vi "DAQmxDigitalOutput_2019-11-01.vi"() -> ()   [LabVIEW 2015]
uses:
  <vilib>/Analysis/baseanly.llb/Mean (DBL).vi
  <vilib>/DAQmx/create/channels.llb/DAQmx Create Channel (CO-Pulse Generation-Time).vi
  <vilib>/DAQmx/configure/timing.llb/DAQmx Timing (Implicit).vi
  MVCAMSDK.dll
  <vilib>/Analysis/NI_AALBase.lvlib
  <vilib>/Analysis/NI_AAL_SigProc.lvlib
panel:
  out "相对误差":dbl=0.8988653041973323
  out "mean":dbl=15.208009079636986 caption="泰伯距离均值Z" format="%0.2f"
  in  "光栅常数d":dbl=0.09854
  in  "error in 2":errorcluster caption="错误输入"
  in  "data 2":bool[](array[boolean])=[TRUE]
  out "测量得到的波长":dbl=638.4880196449607
  out "泰伯距离数值":dbl[](array[numeric])=[15.393849374426454, 15.239052716055017, 15.197063981826837, 15.002070246239633]
  out "移动次数":dbl=1.0
  out "Locations":dbl[](array[numeric])=[10.438621227921368, 25.832470602347822, 41.07152331840284, 56.268587300229676, 71.27065754646931] caption="上面图像曲线波峰位置"
  out "光强图":u8[](graph)=[255, 255, 255, 255, 255, 255, 255, 255, 255, 154, 43, 20, 23, 22, 53, 146, 167, 169, 232, 255, 255, 255, 255, 255, 203, 166, 115, 72, 50, 24, 17, 38, 118, 114, 190, 255, 255, 255, 255, 255, 255, 255, 255, 233, 255, 216, 118, 34, 16, 17, 18, 55, 150, 246, 222, 224, 255, 255, 255, 255, 255, 255, 150, 104, 77, 71, 41, 22, 45, 119, 116, 218, 255, 255, 255, 255, 255, 255, 255, 255, 241, 255, 255, 174, 87, 33, 17, 18, 43, 114, 155, 143, 170, 255, 255, 255, 255, 255, 255, 198, 155, 125, 91, 53, 22, 27, 94, 64, 126, 248, 255, 255, 255, 255, 255, 255, 255, 238, 232, 255, 240, 144, 46, 22, 19, 23, 66, 147, 147, 141, 229, 255, 255, 255, 255, 255, 213, 193, 158, 137, 76, 31, 26, 43, 38, 88, 233, 255, 255, 255, 255, 255, 255, 255, 255, 255, 255, 255, 210, 82, 24, 16, 18, 38, 90, 113, 91, 121, 255, 255, 255, 255, 255, 255, 213, 204, 134, 103, 66, 48, 32, 33, 60, 185, 249, 255, 255, 255, 255, 255, 255, 255, 255, 255, 255, 228, 114, 53, 26, 20, 21, 61, 114, 122, 134, 255, 255, 255, 255, 255, 223, 157, 157, 110, 82, 71, 43, 42, 41, 75, 184, 255, 255, 255, 255, 255, 255, 255, 255, 255, 255, 255, 255, 129, 45, 20, 22, 19, 46, 110, 123, 156, 245, 255, 255, 255, 255, 255, 156, 140, 99, 60, 90, 47, 41, 54, 47, 117, 189, 226, 204, 211, 255, 255, 255, 255, 255, 255, 255, 224, 129, 49, 21, 17, 20, 42, 116, 152, 141, 178, 255, 255, 255, 255, 255, 233, 146, 115, 58, 85, 50, 36, 31, 36, 109, 200, 227, 192, 178, 255, 255, 255, 255, 255, 255, 236, 216, 146, 71, 23, 34, 55, 48, 84, 126, 110, 122, 208, 255, 255, 255, 255, 196, 98, 66, 41, 74, 47, 29, 25, 34, 100, 194, 255, 247, 200, 255, 255, 255, 255, 255, 245, 181, 167, 138, 82, 38, 24, 31, 38, 59, 100, 107, 122, 228, 255, 255, 255, 255, 255, 183, 109, 56, 72, 61, 31, 23, 18, 39, 134, 220, 207, 162, 213, 255, 255, 255, 255, 255, 206, 192, 163, 108, 51, 22, 27, 31, 60, 94, 122, 117, 149, 255, 255, 255, 255, 255, 255, 254, 111]
  out "找到的波谷":i32=5
  out "找到的波峰":i32=5
  out "信号曲线":cluster{"Locations":dbl[], "Amplitudes":dbl[]}[](graph)=[{"Locations"=array[750 elements], "Amplitudes"=array[749 elements]}, {"Locations"=[104.38621227921368, 258.3247060234782, 410.71523318402836, 562.6858730022967, 712.7065754646931], "Amplitudes"=[11153.698204083417, 10559.387052180104, 10974.865031894917, 10500.852817232146, 11059.763900010517]}, {"Locations"=[26.787398227992274, 182.39455189327623, 333.5517219531509, 488.1851999460032, 636.5270621135614], "Amplitudes"=[3284.809720018355, 2039.4564261182056, 3638.2587716464914, 3082.2730888167225, 4217.856016996603]}]
  in  "波峰检测器宽度":i32=5 min=3
  out "相机每次行进距离":dbl=0.1 format="%.2f"
  in  "error in":errorcluster caption="错误输入"
  in  "单次输入步进电机脉冲数":i32=20
  in  "data":bool[](array[boolean])=[FALSE]
  in  "开始测量":bool
  out "相机图像":T1(plugin-control)
  in  "读取自定义数据":bool
  out "从相机1中读出的字符串(32字节)":string
  in  "写入自定义数据":bool
  in  "要写入相机1的字符串(32字节)":string
  in  "拍照":bool
  in  "显示相机参数面板":bool
  in  "Stop":bool
  in  "?":bool
  # "mm"
  # "理论值632.8nm"
  # "%"
  # "mm"
  # "mm"
  # "用泰伯效应测量632.8nm激光波长"
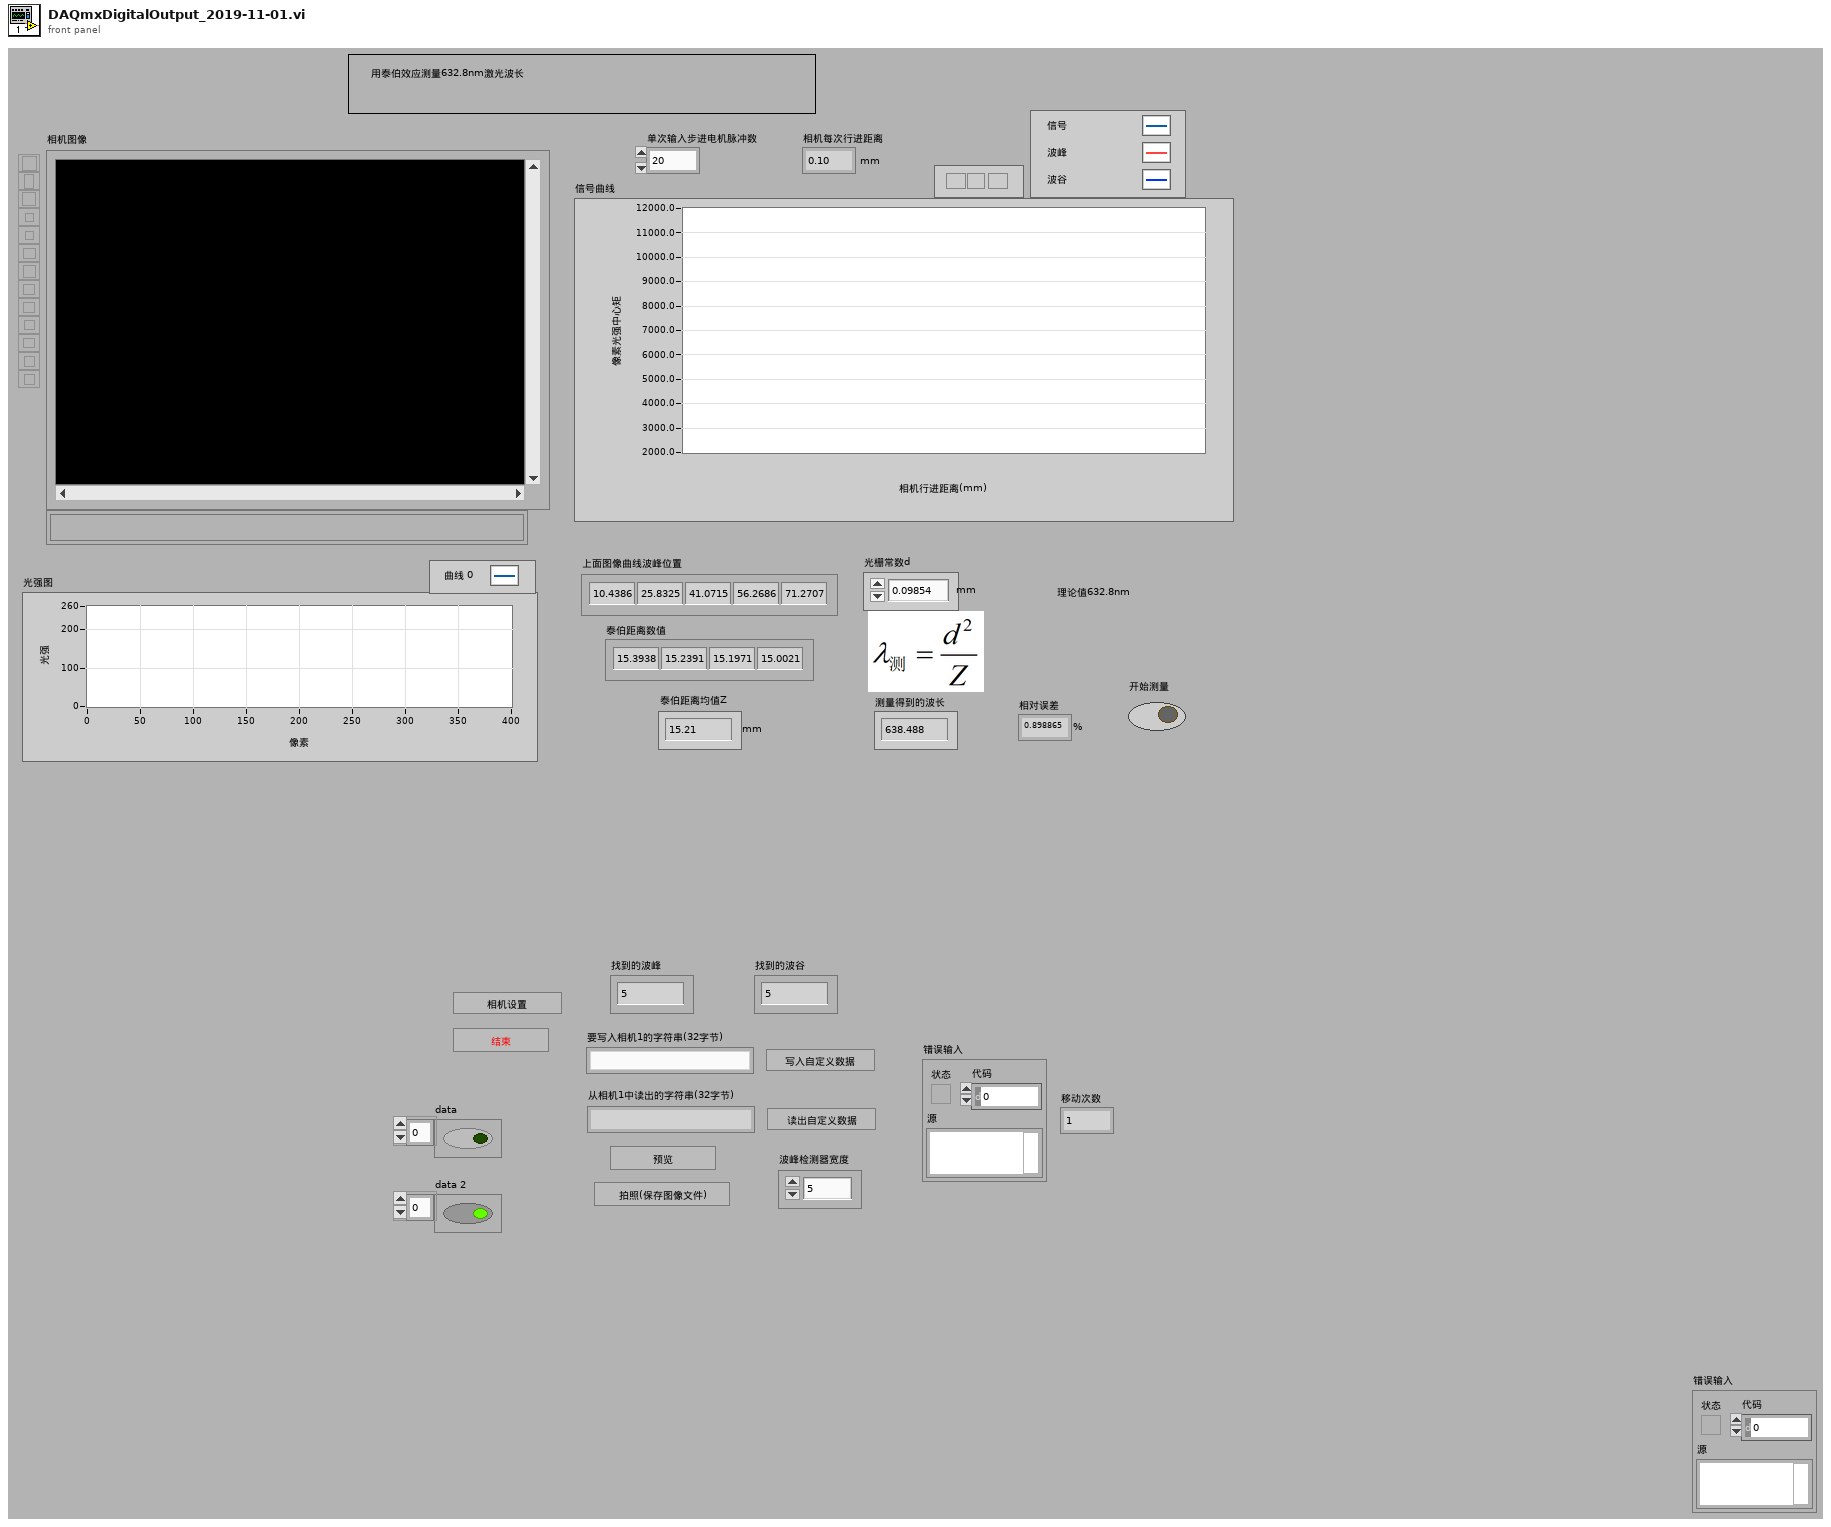
[diagram p1: front panel]
types:
  T1 = typedef "IMAQ Image.ctl" = refnum<image>
  T2 = typedef "Image Type" = u32
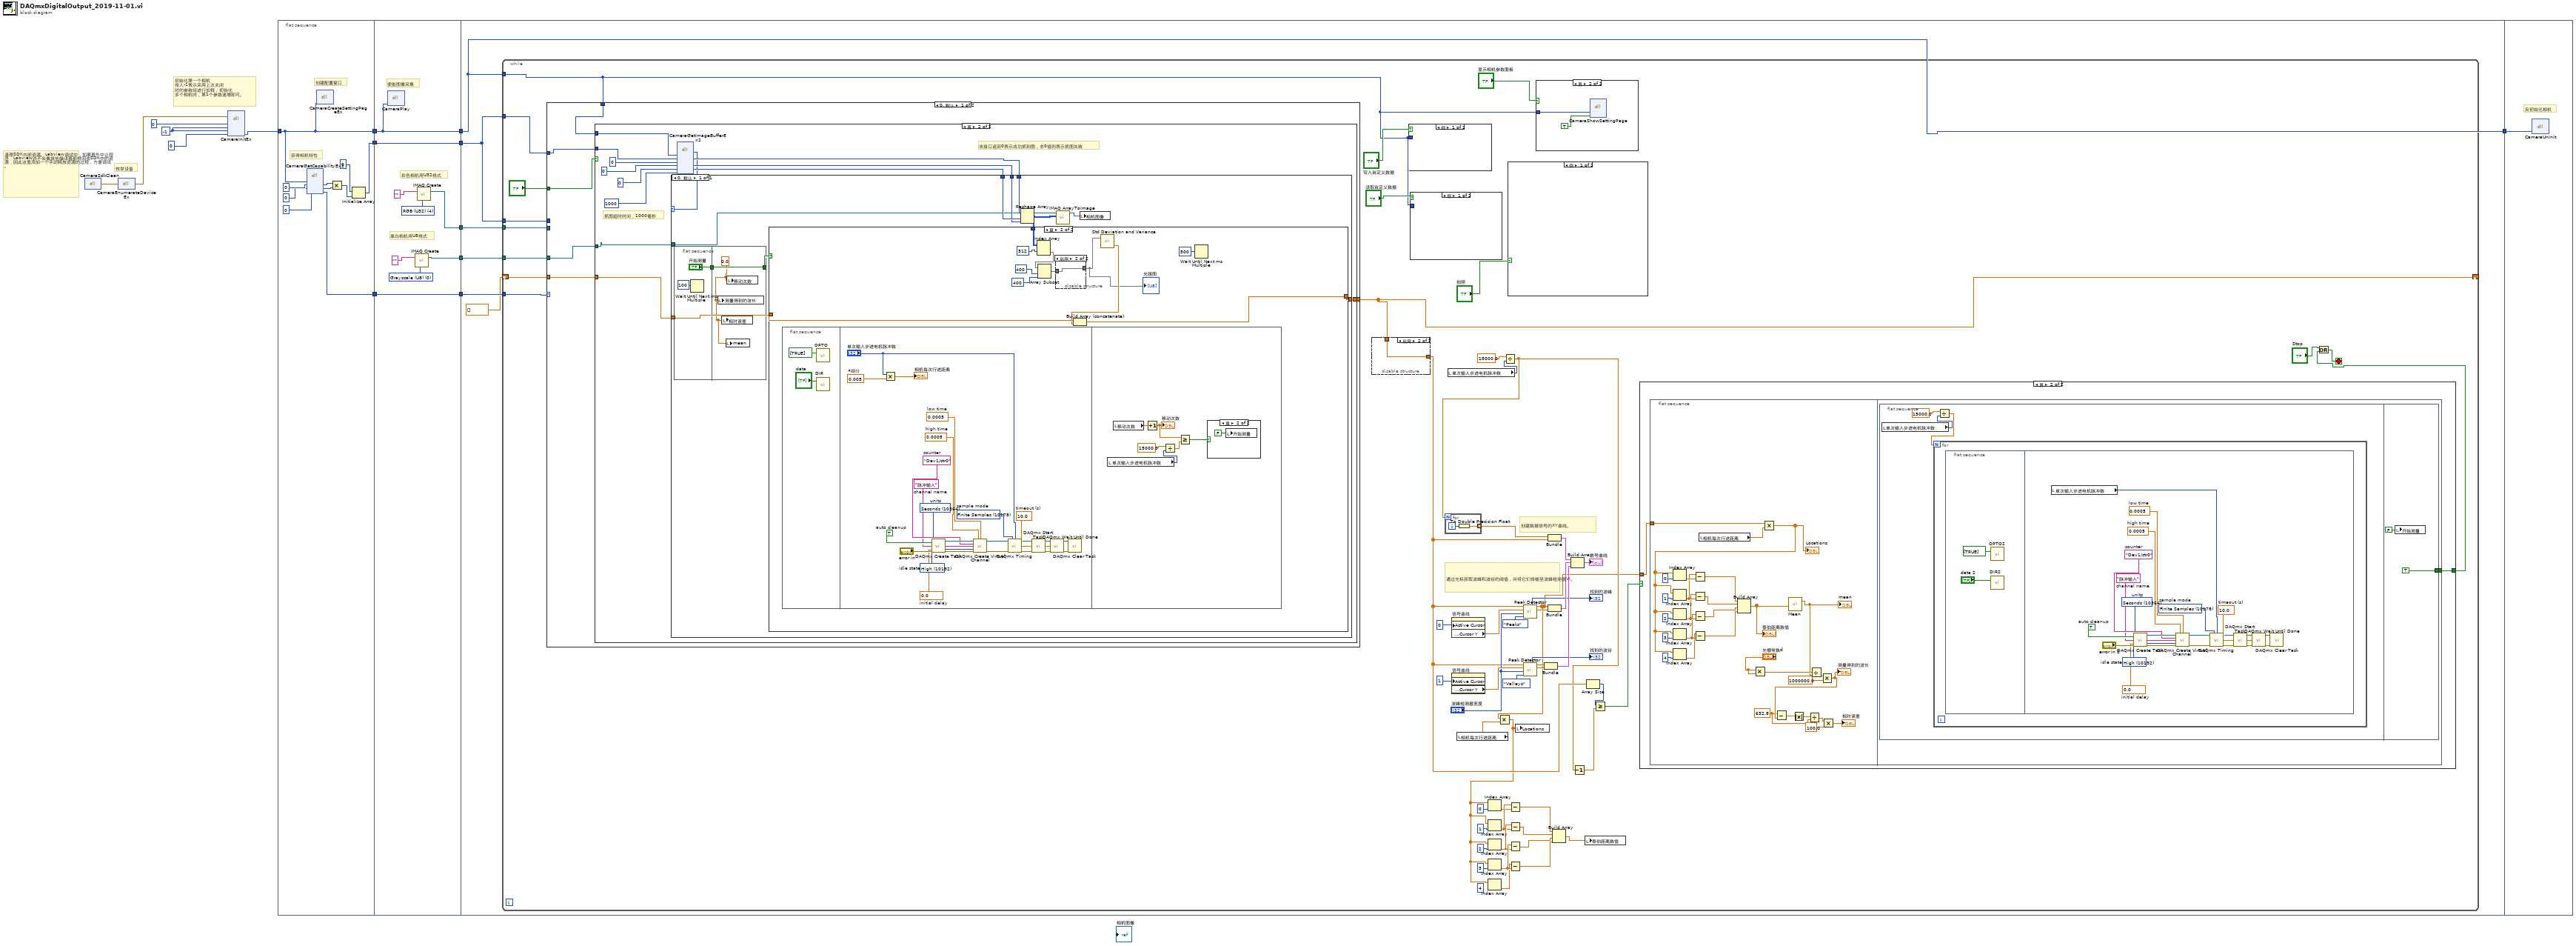
[diagram p0: block diagram]
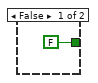
[diagram p2: hidden frame]
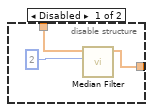
[diagram p3: hidden frame]
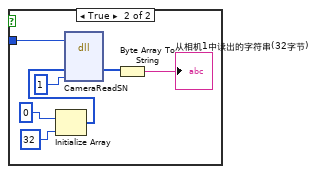
[diagram p4: hidden frame]
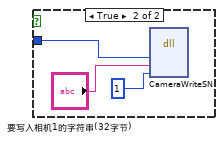
[diagram p5: hidden frame]
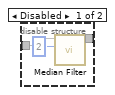
[diagram p8: hidden frame]
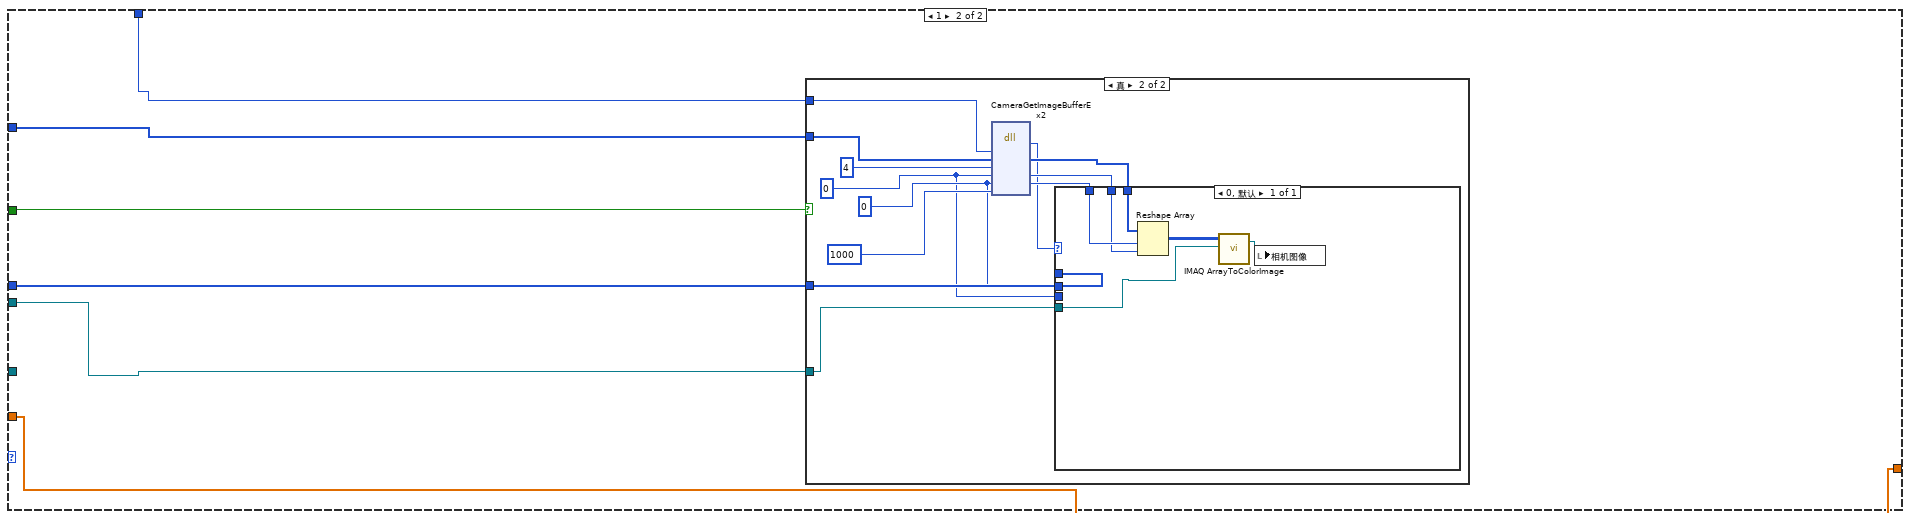
[diagram p10: hidden frame]
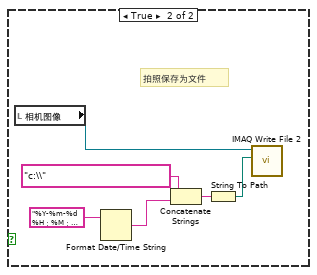
[diagram p12: hidden frame]
diagram:
  w3 = -1
  # "枚举设备"
  # "初始化第一个相机\n传入-1表示采用上次关闭\n时的参数组进行加载；初始化\n多个相机时，第1个参数递增即可。"
  # "清理SDK内部资源。Labview调试中，如果意外中止程序，Labview并不会像其他编译器那样回收SDK中的资源，因此这里添加一个手动释放资源的过程，方便调试。"
  n1 = dll-call lib="MVCAMSDK.dll" fn="CameraSdkClean"() -> (error out=w6:errorcluster)  [unwired: 4 in, 1 out]
  n2 = dll-call lib="MVCAMSDK.dll" fn="CameraEnumerateDeviceEx"(error in=w6) -> (error out=w1:errorcluster)  [unwired: 3 in, 1 out]
  n3 = dll-call lib="MVCAMSDK.dll" fn="CameraInitEx"(error in=w1, "相机索引值"=0, "参数加载方式"=w3, "要加载的参数组索引"=w3, "相机句柄"=0) -> ("相机句柄"=w2:i32)  [unwired: 6 in, 2 out]
  n4 = flat-sequence {
    tunnel: [w16] -> w12
    tunnel: [w23] -> w11
    tunnel: [w17] -> w9
    tunnel: w2 -> [w16]
    tunnel: w12 -> [w34]
    tunnel: [w34] -> w15
    tunnel: [w31] -> w13
    tunnel: w11 -> [w30]
    tunnel: [w30] -> w10
    tunnel: w9 -> [w29]
    tunnel: [w29] -> w8
    tunnel: [w26] -> w7
    tunnel: w15 -> [w38]
    tunnel: [w38] -> w14
    tunnel: w13 -> [w40]
    tunnel: w10 -> [w36]
    tunnel: w8 -> [w39]
    tunnel: w7 -> [w37]
    tunnel: w14 -> [w292]
    frame #0 {
      # "获得相机特性"
      # "创建配置窗口"
      n5 = dll-call lib="MVCAMSDK.dll" fn="CameraGetCapabilityEx2"("相机句柄"=w16, "图像最大宽度"=0, "图像最大高度"=0, "是否是彩色相机(返回0:黑白;1:彩色)"=0) -> ("图像最大宽度"=w19:i32, "图像最大高度"=w18:i32, "是否是彩色相机(返回0:黑白;1:彩色)"=w17:i32)  [unwired: 5 in, 2 out]
      n6 = dll-call lib="MVCAMSDK.dll" fn="CameraCreateSettingPageEx"("相机句柄"=w16) -> ()  [unwired: 5 in, 2 out]
      n7 = Multiply(x=w19, y=w18) -> (x*y=w24:i32)
      n8 = Initialize Array(0, w24) -> (w23:i32[])
    }
    frame #1 {
      w28 = T2 0 items=["Grayscale (U8)", "Grayscale (I16)", "Grayscale (SGL)", "Complex (CSG)", "RGB (U32)", "HSL (U32)", "RGB (U64)", "Grayscale (U16)"] ("Image Type")
      w33 = T2 4 items=["Grayscale (U8)", "Grayscale (I16)", "Grayscale (SGL)", "Complex (CSG)", "RGB (U32)", "HSL (U32)", "RGB (U64)", "Grayscale (U16)"] ("Image Type")
      # "黑白相机用U8格式"
      # "彩色相机用U32格式"
      # "使能图像采集"
      n9 = dll-call lib="MVCAMSDK.dll" fn="CameraPlay"("相机句柄"=w34) -> ()  [unwired: 5 in, 2 out]
      n10 = call "IMAQ Create"("Image Name"="", "Image Type"=w28) -> ("New Image"=w26:T1)  [unwired: 3 in, 1 out]
      n11 = call "IMAQ Create"("Image Name"="", "Image Type"=w33) -> ("New Image"=w31:T1)  [unwired: 3 in, 1 out]
    }
    frame #2 {
      n12 = while {
        tunnel: w38 -> [w87]
        tunnel: w40 -> [w94]
        tunnel: w36 -> [w95]
        tunnel: w39 -> [w93]
        tunnel: w37 -> [w91]
        tunnel: w36 -> [w90]
        shift-right: [w85] -> _
        shift-left: dbl[] [] -> [w86]
        stop <- w58 stop-if-true
        (unwired) 4 ("索引")
        # "通过光标获取波峰和波谷的阈值，并将它们传输至波峰检测器VI。"
        # "创建数据信号的XY曲线。"
        n13 = case shown="0, 默认" w93 {
          tunnel: w95 -> [w180 w265]
          tunnel: w94 -> [_ w262]
          tunnel: w87 -> [w181 w264]
          tunnel: "?" -> [w179 w263]
          tunnel: w91 -> [w182 _]
          tunnel: w90 -> [_ w261]
          tunnel: w86 -> [w178 w260]
          tunnel: [w177 w260] -> w85
          frame 0, Default {
            n14 = case shown="真" w179 {
              tunnel: w181 -> [_ w196]
              tunnel: w180 -> [_ w187]
              tunnel: w182 -> [_ w186]
              tunnel: w178 -> [w183 w185]
              tunnel: [w183 w184] -> w177
              frame False {
              }
              frame True {
                # "该接口返回0表示成功抓到图，非0值则表示抓图失败"
                # "抓图超时时间，1000毫秒"
                n15 = dll-call lib="MVCAMSDK.dll" fn="CameraGetImageBufferEx2"("相机句柄"=w196, "图像数据缓冲区"=w187, "图像输出格式(0:8位灰度;1:24位彩色;2:32位彩色)"=0, "图像宽度"=0, "图像高度"=0, "抓图超时时间(毫秒)"=1000) -> ("返回类型"=w188:i32, "图像数据缓冲区"=w191:u8[], "图像宽度"=w189:i32, "图像高度"=w190:i32)  [unwired: 6 in, 2 out]
                n16 = case shown="0, 默认" w188 {
                  tunnel: w191 -> [w206]
                  tunnel: w186 -> [w203]
                  tunnel: w190 -> [w205]
                  tunnel: w189 -> [w204]
                  tunnel: w185 -> [w199]
                  tunnel: [w198] -> w184
                  frame 0, Default {
                    n17 = flat-sequence {
                      tunnel: ["开始测量"] -> w197
                      tunnel: [w210] -> w200
                      tunnel: w197 -> [w210]
                      frame #0 {
                        n18 = Wait Until Next ms Multiple(millisecond multiple=u32 100 ("毫秒倍数")) -> ()  [unwired: 1 out]
                      }
                      frame #1 {
                        w209 = 0.0 ("移动次数")
                        n19 = local write "测量得到的波长"(w209) -> ()
                        n20 = local write "相对误差"(w209) -> ()
                        n21 = local write "mean"(w209) -> ()
                        n22 = local write "移动次数"(w209) -> ()
                      }
                    }
                    n23 = Reshape Array(w206, w205, w204) -> (w201:u8[][])
                    n24 = case shown="真" w200 {
                      tunnel: w201 -> [_ w222]
                      tunnel: w199 -> [w211 w216]
                      tunnel: [w211 w215] -> w198
                      frame False {
                      }
                      frame True {
                        n25 = flat-sequence {
                          frame #0 {
                            n26 = call "OPTO"("data"=bool[] [TRUE]) -> ()  [unwired: 17 in, 2 out]
                            n27 = call "DIR"("data"="data") -> ()  [unwired: 17 in, 2 out]
                          }
                          frame #1 {
                            w230 = 0.005  # 4细分
                            w234 = 10178 items=["Finite Samples"=10178, "Continuous Samples"=10123, "Hardware Timed Single Point"=12522]  # sample mode
                            w236 = 0.0005  # low time
                            w237 = 0.0005  # high time
                            w238 = 0.0  # initial delay
                            w239 = 10192 items=["High"=10192, "Low"=10214]  # idle state
                            w240 = 10364 items=["Seconds"=10364, "From Custom Scale"=10065]  # units
                            w241 = "脉冲输入"  # channel name
                            w243 = "Dev1/ctr0"  # counter
                            w245 = TRUE  # auto cleanup
                            w249 = 10.0  # timeout (s)
                            n28 = Multiply(x="单次输入步进电机脉冲数", y=w230) -> (x*y=→"相机每次行进距离":dbl)
                            n29 = call <vilib>:"DAQmx Create Task.vi"("auto cleanup"=w245, "error in"="error in") -> ("task out"=w244:refnum<k21>, "error out"=w246:errorcluster)  [unwired: 12 in]
                            n30 = call-poly <vilib>:"DAQmx Create Virtual Channel.vi"("task in"=w244, "high time"=w237, "low time"=w236, "counter"=w243, "name to assign"=w241, "units"=w240, "error in"=w246, "idle state"=w239, "initial delay"=w238) -> ("task out"=w235:refnum<k21>, "error out"=w242:errorcluster)  [unwired: 5 in]
                            n31 = call-poly <vilib>:"DAQmx Timing.vi"("task/channels in"=w235, "sample mode"=w234, "samples per channel"="单次输入步进电机脉冲数", "error in"=w242) -> ("task out"=w233:refnum<k21>, "error out"=w232:errorcluster)  [unwired: 10 in]
                            n32 = call <vilib>:"DAQmx Start Task.vi"("task/channels in"=w233, "error in"=w232) -> ("task out"=w252:refnum<k21>, "error out"=w251:errorcluster)  [unwired: 12 in]
                            n33 = call <vilib>:"DAQmx Wait Until Done.vi"("task/channels in"=w252, "timeout (sec)"=w249, "error in"=w251) -> ("task out"=w248:refnum<k21>, "error out"=w250:errorcluster)  [unwired: 11 in]
                            n34 = call <vilib>:"DAQmx Clear Task.vi"("task in"=w248, "error in"=w250) -> ()  [unwired: 13 in, 1 out]
                          }
                          frame #2 {
                            n35 = local read "单次输入步进电机脉冲数"() -> (w254:i32)
                            n36 = local read "移动次数"() -> (w258:dbl)
                            n37 = Increment(x=w258) -> (x+1=w257:dbl)
                            "移动次数" <- w257
                            n38 = Divide(x=15000.0 ("y"), y=w254) -> (x/y=w253:dbl)
                            n39 = Greater Or Equal?(x=w257, y=w253) -> (x >= y?=w256:bool)
                            n40 = case shown="真" w256 {
                              frame False {
                              }
                              frame True {
                                n41 = local write "开始测量"(FALSE ("开始测量")) -> ()
                              }
                            }
                          }
                        }
                        n42 = Index Array(array=w222, index (row)=512 ("索引 (行)")) -> (element=w220:u8[])  [unwired: 1 in]
                        n43 = Array Subset(array=w220, index=400 ("索引"), length=400 ("长度")) -> (w218:u8[])
                        n44 = disable-structure shown="启用" {
                          disable-tunnel: w218 -> [w225 w226]
                          disable-tunnel: [w223 w226] -> w212
                          frame Disabled {
                            n45 = call <vilib>:"Median Filter.vi"("left rank"=2, "X"=w225) -> ("Filtered X"=w223:dbl[])  [unwired: 8 in, 1 out]
                          }
                          frame Enabled {
                          }
                        }
                        "光强图" <- w212
                        n46 = call <vilib>:"Std Deviation and Variance.vi"("X"=w212) -> ("variance"=w213:dbl)  [unwired: 1 in, 2 out]
                        n47 = Build Array (concatenate)(w216, w213) -> (w215:dbl[])
                        n48 = Wait Until Next ms Multiple(millisecond multiple=u32 500 ("毫秒倍数")) -> ()  [unwired: 1 out]
                      }
                    }
                    n49 = call "IMAQ ArrayToImage"("Image Pixels (U8)"=w201, "Image"=w203) -> ("Image Out"=w202:T1)  [unwired: 8 in, 1 out]
                    n50 = local write "相机图像"(w202) -> ()
                  }
                }
              }
            }
          }
          frame 1 {
            n51 = case shown="真" w263 {
              tunnel: w264 -> [_ w277]
              tunnel: w262 -> [_ w270]
              tunnel: w265 -> [_ w269]
              tunnel: w261 -> [_ w268]
              frame False {
              }
              frame True {
                w266 = 0
                w267 = 0
                n52 = dll-call lib="MVCAMSDK.dll" fn="CameraGetImageBufferEx2"("相机句柄"=w277, "图像数据缓冲区"=w269, "图像输出格式(0:8位灰度;1:24位彩色;2:32位彩色)"=4, "图像宽度"=w266, "图像高度"=w267, "抓图超时时间(毫秒)"=1000) -> ("返回类型"=w271:i32, "图像数据缓冲区"=w274:u32[], "图像宽度"=w272:i32, "图像高度"=w273:i32)  [unwired: 6 in, 2 out]
                n53 = case shown="0, 默认" w271 {
                  tunnel: w274 -> [w283]
                  tunnel: w270 -> [w279]
                  tunnel: w273 -> [w282]
                  tunnel: w272 -> [w281]
                  tunnel: w268 -> [_]
                  tunnel: w267 -> [_]
                  tunnel: w266 -> [_]
                  frame 0, Default {
                    n54 = Reshape Array(w283, w282, w281) -> (w278:u32[][])
                    n55 = call "IMAQ ArrayToColorImage"("Image Pixels (U32)"=w278, "Image"=w279) -> ("Image Out"=w280:T1)  [unwired: 3 in, 1 out]
                    n56 = local write "相机图像"(w280) -> ()
                  }
                }
              }
            }
          }
        }
        n57 = disable-structure shown="启用" {
          disable-tunnel: w85 -> [w164 w166]
          disable-tunnel: [w163 w166] -> w67
          frame Disabled {
            n58 = call <vilib>:"Median Filter.vi"("left rank"=2, "X"=w164) -> ("Filtered X"=w163:dbl[])  [unwired: 8 in, 1 out]
          }
          frame Enabled {
          }
        }
        n59 = case shown="假" "写入自定义数据" {
          tunnel: w87 -> [_ w176]
          frame False {
          }
          frame True {
            n60 = dll-call lib="MVCAMSDK.dll" fn="CameraWriteSN"("相机句柄"=w176, "序列号(固定为32个字节)"="要写入相机1的字符串(32字节)", "序列号级别，[0,1,2]对应3级序列号，其中0级为只读，1,2级可写"=1) -> ()  [unwired: 7 in, 2 out]
          }
        }
        n61 = case shown="假" "读取自定义数据" {
          tunnel: w87 -> [_ w173]
          frame False {
          }
          frame True {
            n62 = Initialize Array(0, 32) -> (w170:i32[])
            n63 = dll-call lib="MVCAMSDK.dll" fn="CameraReadSN"("相机句柄"=w173, "序列号"=w170, "序列号级别，[0,1,2],0级为只读，1,2级可写"=1) -> ("序列号"=w168:u8[])  [unwired: 6 in, 2 out]
            n64 = Byte Array To String(unsigned byte array=w168) -> (string=→"从相机1中读出的字符串(32字节)":string)
          }
        }
        n65 = local read "单次输入步进电机脉冲数"() -> (w64:i32)
        n66 = property on="信号曲线" class="XYGraph (严格)"("Active Cursor"=u32 0) -> ("Cursor.Cursor Position:Cursor Y"=w74:dbl)  [unwired: 2 in, 2 out]
        n67 = property on="信号曲线" class="XYGraph (严格)"("Active Cursor"=u32 1) -> ("Cursor.Cursor Position:Cursor Y"=w73:dbl)  [unwired: 2 in, 2 out]
        n68 = local read "相机每次行进距离"() -> (w57:dbl)
        n69 = Divide(x=15000.0 ("y"), y=w64) -> (x/y=w61:dbl)
        n70 = for {
          N: w61 -> [_]
          tunnel: [w161] -> w75 mode=indexing
          i -> [w162]
          n71 = To Double Precision Float(number=w162) -> (double precision float=w161:dbl)
        }
        n72 = case shown="假" "拍照" {
          frame False {
          }
          frame True {
            # "拍照保存为文件"
            n73 = local read "相机图像"() -> (w284:T1)
            n74 = Format Date/Time String(time format string (%c)="%Y-%m-%d %H：%M：%S.bmp ") -> (date/time string=w288:string)  [unwired: 2 in]
            n75 = Concatenate Strings("c:\\", w288) -> (w285:string)
            n76 = String To Path(string=w285) -> (path=w287:path)
            n77 = call-poly "IMAQ Write File 2"("File Path"=w287, "Image"=w284) -> ()  [unwired: 8 in, 2 out]
          }
        }
        n78 = call <vilib>:"Peak Detector.vi"("peaks/valleys"=enum32{"Peaks", "Valleys"}."Peaks", "width"="波峰检测器宽度", "threshold"=w74, "X"=w67) -> ("Amplitudes"=w82:dbl[], "Locations"=w56:dbl[], "# found"=→"找到的波峰":i32)  [unwired: 3 in, 2 out]
        n79 = Multiply(x=w56, y=w57) -> (x*y=w43:dbl[])
        n80 = Index Array(array=w43, index=0 ("索引")) -> (element=w48:dbl)
        n81 = Index Array(array=w43, index=1 ("索引")) -> (element=w49:dbl)
        n82 = Index Array(array=w43, index=2 ("索引")) -> (element=w50:dbl)
        n83 = Index Array(array=w43, index=3 ("索引")) -> (element=w51:dbl)
        n84 = Index Array(array=w43) -> (element=w41:dbl)  [unwired: 1 in]
        n85 = Subtract(x=w49, y=w48) -> (x-y=w52:dbl)
        n86 = Subtract(x=w50, y=w49) -> (x-y=w53:dbl)
        n87 = Subtract(x=w51, y=w50) -> (x-y=w54:dbl)
        n88 = Subtract(x=w41, y=w51) -> (x-y=w55:dbl)
        n89 = local write "Locations"(w43) -> ()
        n90 = call <vilib>:"Peak Detector.vi"("peaks/valleys"=enum32{"Peaks", "Valleys"}."Valleys", "width"="波峰检测器宽度", "threshold"=w73, "X"=w67) -> ("Amplitudes"=w79:dbl[], "Locations"=w80:dbl[], "# found"=→"找到的波谷":i32)  [unwired: 3 in, 2 out]
        n91 = case shown="真" "显示相机参数面板" {
          tunnel: w87 -> [_ w291]
          frame False {
          }
          frame True {
            n92 = dll-call lib="MVCAMSDK.dll" fn="CameraShowSettingPage"("相机句柄"=w291, "状态"=TRUE) -> ()  [unwired: 6 in, 2 out]
          }
        }
        n93 = Bundle("Locations"=w80, "Amplitudes"=w79) -> (w77:cluster{"Locations":dbl[], "Amplitudes":dbl[]})  [unwired: 1 in]
        n94 = Bundle(w75, w67) -> (w84:cluster{dbl[], dbl[]})  [unwired: 1 in]
        n95 = Bundle("Locations"=w56, "Amplitudes"=w82) -> (w81:cluster{"Locations":dbl[], "Amplitudes":dbl[]})  [unwired: 1 in]
        n96 = Build Array(w52, w53, w54, w55) -> (w42:dbl[])
        n97 = Build Array(w84, w81, w77) -> (→"信号曲线":cluster{"Locations":dbl[], "Amplitudes":dbl[]}[])
        n98 = Decrement(x=w61) -> (x-1=w62:dbl)
        n99 = local write "泰伯距离数值"(w42) -> ()
        n100 = Array Size(array=w67) -> (size(s)=w66:i32)
        n101 = Greater Or Equal?(x=w66, y=w62) -> (x >= y?=w65:bool)
        n102 = case shown="真" w65 {
          tunnel: w56 -> [_ w100]
          tunnel: [FALSE w99] -> w59
          frame False {
          }
          frame True {
            n103 = flat-sequence {
              tunnel: w100 -> [w116]
              tunnel: [w131] -> w99
              frame #0 {
                w105 = 632.8 ("x")
                n104 = local read "相机每次行进距离"() -> (w111:dbl)
                n105 = Multiply(x="光栅常数d", y="光栅常数d") -> (x*y=w113:dbl)
                n106 = Multiply(x=w116, y=w111) -> (x*y=w115:dbl[])
                "Locations" <- w115
                n107 = Index Array(array=w115, index=0 ("索引")) -> (element=w125:dbl)
                n108 = Index Array(array=w115, index=1 ("索引")) -> (element=w124:dbl)
                n109 = Index Array(array=w115, index=2 ("索引")) -> (element=w123:dbl)
                n110 = Index Array(array=w115, index=3 ("索引")) -> (element=w122:dbl)
                n111 = Index Array(array=w115, index=4 ("索引")) -> (element=w121:dbl)
                n112 = Subtract(x=w124, y=w125) -> (x-y=w120:dbl)
                n113 = Subtract(x=w123, y=w124) -> (x-y=w119:dbl)
                n114 = Subtract(x=w122, y=w123) -> (x-y=w118:dbl)
                n115 = Subtract(x=w121, y=w122) -> (x-y=w117:dbl)
                n116 = Build Array(w120, w119, w118, w117) -> (w101:dbl[])
                "泰伯距离数值" <- w101
                n117 = call-poly <vilib>:"Mean.vi"("X"=w101) -> ("mean"=w112:dbl)  [unwired: 1 out]
                "mean" <- w112
                n118 = Divide(x=w113, y=w112) -> (x/y=w110:dbl)
                n119 = Multiply(x=w110, y=1000000.0) -> (x*y=w108:dbl)
                "测量得到的波长" <- w108
                n120 = Subtract(x=w105, y=w108) -> (x-y=w107:dbl)
                n121 = Absolute Value(x=w107) -> (abs(x)=w106:dbl)
                n122 = Divide(x=w106, y=w105) -> (x/y=w104:dbl)
                n123 = Multiply(x=w104, y=100.0) -> (x*y=→"相对误差":dbl)
              }
              frame #1 {
                n124 = flat-sequence {
                  tunnel: [TRUE] -> w131
                  frame #0 {
                    n125 = local read "单次输入步进电机脉冲数"() -> (w133:i32)
                    n126 = Divide(x=15000.0 ("y"), y=w133) -> (x/y=w132:dbl)
                    n127 = for {
                      N: w132 -> [_]
                      n128 = flat-sequence {
                        frame #0 {
                          n129 = call "OPTO2"("data"=bool[] [TRUE]) -> ()  [unwired: 17 in, 2 out]
                          n130 = call "DIR2"("data"="data 2") -> ()  [unwired: 17 in, 2 out]
                        }
                        frame #1 {
                          w140 = 10178 items=["Finite Samples"=10178, "Continuous Samples"=10123, "Hardware Timed Single Point"=12522]  # sample mode
                          w142 = 0.0005  # low time
                          w143 = 0.0005  # high time
                          w144 = 0.0  # initial delay
                          w145 = 10192 items=["High"=10192, "Low"=10214]  # idle state
                          w146 = 10364 items=["Seconds"=10364, "From Custom Scale"=10065]  # units
                          w147 = "脉冲输入"  # channel name
                          w149 = "Dev1/ctr0"  # counter
                          w151 = TRUE  # auto cleanup
                          w155 = 10.0  # timeout (s)
                          n131 = local read "单次输入步进电机脉冲数"() -> (w137:i32)
                          n132 = call <vilib>:"DAQmx Create Task.vi"("auto cleanup"=w151, "error in"="error in 2") -> ("task out"=w150:refnum<k21>, "error out"=w152:errorcluster)  [unwired: 12 in]
                          n133 = call-poly <vilib>:"DAQmx Create Virtual Channel.vi"("task in"=w150, "high time"=w143, "low time"=w142, "counter"=w149, "name to assign"=w147, "units"=w146, "error in"=w152, "idle state"=w145, "initial delay"=w144) -> ("task out"=w141:refnum<k21>, "error out"=w148:errorcluster)  [unwired: 5 in]
                          n134 = call-poly <vilib>:"DAQmx Timing.vi"("task/channels in"=w141, "sample mode"=w140, "samples per channel"=w137, "error in"=w148) -> ("task out"=w139:refnum<k21>, "error out"=w138:errorcluster)  [unwired: 10 in]
                          n135 = call <vilib>:"DAQmx Start Task.vi"("task/channels in"=w139, "error in"=w138) -> ("task out"=w158:refnum<k21>, "error out"=w157:errorcluster)  [unwired: 12 in]
                          n136 = call <vilib>:"DAQmx Wait Until Done.vi"("task/channels in"=w158, "timeout (sec)"=w155, "error in"=w157) -> ("task out"=w154:refnum<k21>, "error out"=w156:errorcluster)  [unwired: 11 in]
                          n137 = call <vilib>:"DAQmx Clear Task.vi"("task in"=w154, "error in"=w156) -> ()  [unwired: 13 in, 1 out]
                        }
                      }
                    }
                  }
                  frame #1 {
                    n138 = local write "开始测量"(FALSE ("开始测量")) -> ()
                  }
                }
              }
            }
          }
        }
        n139 = Or(x="Stop", y=w59) -> (x .or. y?=w58:bool)
      }
    }
    frame #3 {
      # "反初始化相机"
      n140 = dll-call lib="MVCAMSDK.dll" fn="CameraUnInit"("相机句柄"=w292) -> ()  [unwired: 5 in, 2 out]
    }
  }
